vi "myDAQ 2AnalogSensors_DAQAssistant.vi"() -> ()   [LabVIEW 2018]
uses:
  <vilib>/express/express analysis/Spectral/Block/exnSpectralBlock spectral measurements power poly.vi
  <vilib>/express/express analysis/Spectral/Block/exnSpectralBlock spectral measurements power DDT.vi
  <vilib>/express/express analysis/Spectral/XNode/ExpressSpectralMeasurementsBlockNode.xnode
panel:
  out "Decoded string value":string
  out "return value":string
  in  "module path":path
  out "Frequency Max":dbl
  out "Amplitude Max":dbl
  out "Power Spectrum":dynamicdata(graph)
  out "Wave\nRepresentation":dynamicdata(graph)
  out "data":dynamicdata(graph)
  in  "stop (F)":bool
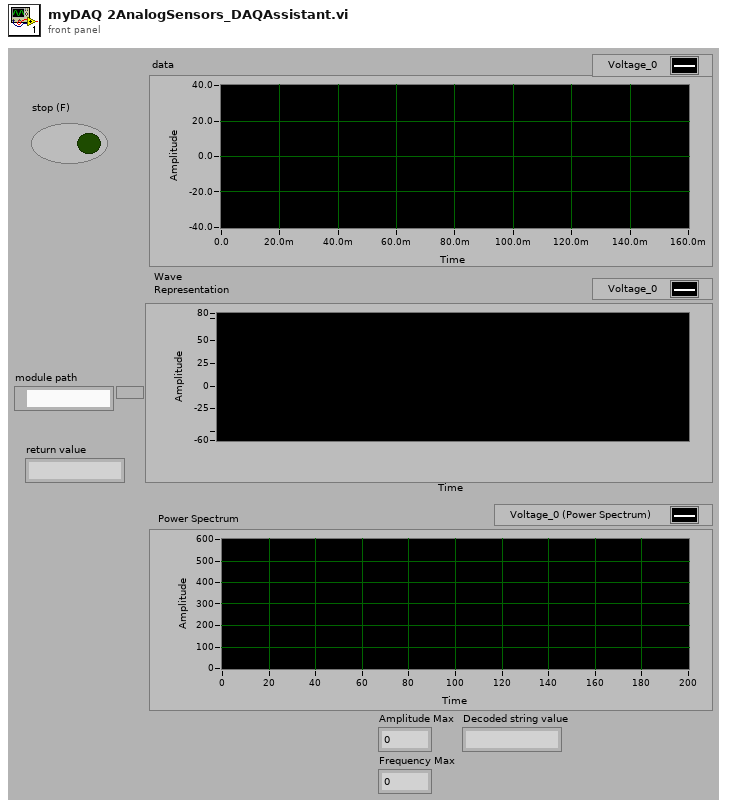
[diagram p1: front panel]
types:
  T1 = cluster{"averaging mode":u16, "weighting mode":u16, "number of averages":u32}
  T2 = cluster{"dB On (F)":bool, "unwrap phase (F)":bool, "convert to degree (F)":bool}
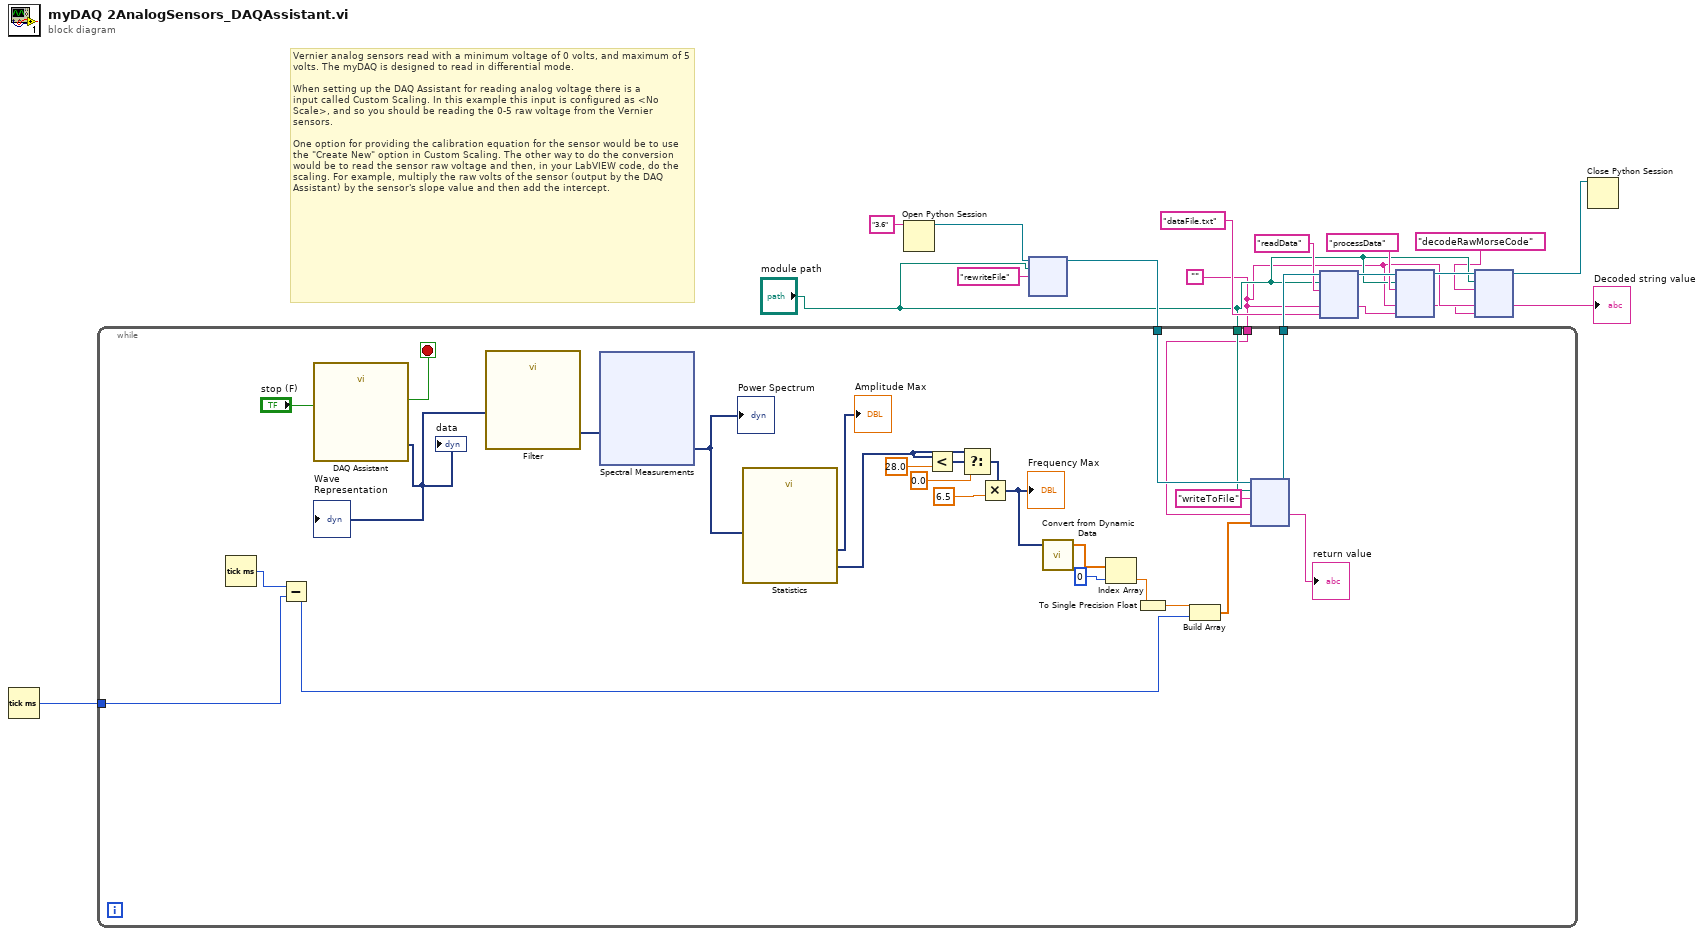
[diagram p0: block diagram]
diagram:
  w3 = ""
  # "Vernier analog sensors read with a minimum voltage of 0 volts, and maximum of 5 volts. The myDAQ is designed to read in differential mode.\n\nWhen setting up the DAQ Assistant for reading analog voltage there is a \ninput called Custom Scaling. In this example this input is configured as <No Scale>, and so you should be reading the 0-5 raw voltage from the Vernier sensors. \n\nOne option for providing the calibration equation for the sensor would be to use the \"Create New\" option in Custom Scaling. The other way to do the conversion would be to read the sensor raw voltage and then, in your LabVIEW code, do the scaling. For example, multiply the raw volts of the sensor (output by the DAQ Assistant) by the sensor's slope value and then add the intercept."
  n1 = Tick Count (ms)() -> (millisecond timer value=w17:u32)
  n2 = Open Python Session(python version="3.6" ("Python version")) -> (session out=w15:refnum<k35>)  [unwired: 2 in, 1 out]
  n3 = node(w15, "module path", "rewriteFile" ("function name")) -> (w14:refnum<k35>)  [unwired: 3 in, 3 out]
  n4 = while {
    tunnel: w14 -> [w32]
    tunnel: [w31] -> w13
    tunnel: "module path" -> [w30]
    tunnel: w17 -> [w25]
    tunnel: w3 -> [w19]
    stop <- w44 stop-if-true
    n5 = Tick Count (ms)() -> (millisecond timer value=w33:u32)
    n6 = Subtract(x=w33, y=w25) -> (x-y=w24:u32)
    n7 = call "DAQ Assistant"("stop (F)"="stop (F)") -> ("data"=w43:dynamicdata, "stopped"=w44:bool)  [unwired: 15 in, 2 out]
    "data" <- w43
    "Wave\nRepresentation" <- w43
    n8 = call "Filter"("Signal"=w43) -> ("Filtered Signal"=w42:dynamicdata)  [unwired: 9 in, 1 out]
    n9 = xnode "Spectral Measurements"("Signals"=w42) -> ("Power Spectrum"=w40:dynamicdata)  [unwired: 1 in, 1 out]
    "Power Spectrum" <- w40
    n10 = call "Statistics"("Signals"=w40) -> ("Index of Max"=w37:dynamicdata, "Maximum"=→"Amplitude Max":dynamicdata)  [unwired: 24 in, 1 out]
    n11 = Less?(x=w37, y=28.0) -> (x < y?=w38:dynamicdata)
    n12 = Select(t=w37, s=w38, f=0.0) -> (s? t:f=w34:dynamicdata)
    n13 = Multiply(x=w34, y=6.5) -> (x*y=w29:dynamicdata)
    "Frequency Max" <- w29
    n14 = call "Convert from Dynamic Data"("Dynamic Data Type"=w29) -> ("Array"=w27:dbl[])  [unwired: 3 in]
    n15 = Index Array(array=w27, index=0) -> (element=w22:dbl)
    n16 = To Single Precision Float(number=w22) -> (single precision float=w21:sgl)
    n17 = Build Array(w21, w24) -> (w23:sgl[])
    n18 = node(w32, w30, "writeToFile" ("function name"), w19, w23) -> (w31:refnum<k35>, →"return value":string)  [unwired: 2 in, 3 out]
  }
  n19 = node(w13, "module path", "readData", w3, "dataFile.txt") -> (w11:refnum<k35>, w2:string)  [unwired: 2 in, 3 out]
  n20 = node(w11, "module path", "processData", w3, w2) -> (w8:refnum<k35>, w1:string)  [unwired: 2 in, 3 out]
  n21 = node(w8, "module path", "decodeRawMorseCode", w3, w1) -> (w4:refnum<k35>, →"Decoded string value":string)  [unwired: 2 in, 3 out]
  n22 = Close Python Session(session in=w4) -> ()  [unwired: 1 in, 1 out]
